vi "PH_SRDG645.evt Call Set Trigger.vi"(0 "i ref in":refnum<vi>, 2 "Generator Instance":string="N/A", 3 "Trigger Settings":T1={"Source"=0, "Rate [Hz]"=1000.0, "Level [V]"=1.0} {"Rate [Hz]" format="%#_9p"; "Source" items=["Internal", "External rising edge", "External falling edge", "Single shot external rising edges", "Single shot external falling edges", "Single shot", "Line"]}, 5 "error IO":errorcluster) -> (14 "i ref out":refnum<vi>, 19 "error out":errorcluster)   [LabVIEW 2014, in "PH_SRDG645.lvlib"]
doc: "This VI sends a simple event call."
uses:
  PH_SRDG645.lvlib
  PH_SRDG645.Trigger.ctl
  CS_Core/CSSystem/CoreLib/CoreLib.int 2 byte array.vi
  CS_Core/CSSystem/CoreLib/CoreLib.double 2 byte array.vi
  CS_Core/CSSystem/CoreLib/CoreLib.lvlib
  CS_Core/BaseProcess/BaseProcess.lvlib
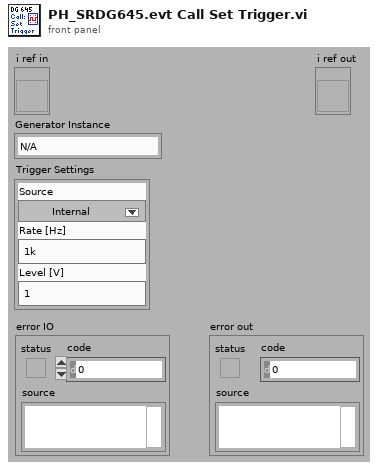
[diagram p1: front panel]
types:
  T1 = typedef "PH_SRDG645.lvlib/PH_SRDG645.Trigger.ctl" = cluster{"Source":i32, "Rate [Hz]":dbl, "Level [V]":dbl}
  T2 = typedef "CoreDefs.rawDataType.ctl" = i8[]
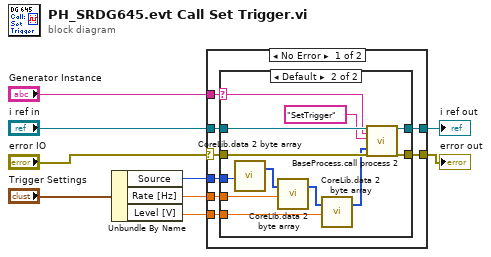
[diagram p0: block diagram]
diagram:
  n1 = Unbundle By Name("Trigger Settings") -> ("Source"=w3:i32, "Rate [Hz]"=w2:dbl, "Level [V]"=w1:dbl)
  n2 = case shown="No Error" "error IO" {
    selector: "error IO" -> [w17 w32]
    tunnel: "Generator Instance" -> [w10 _]
    tunnel: [w16 w32] -> w9
    tunnel: [w14 w33] -> w8
    tunnel: w1 -> [w11 _]
    tunnel: w2 -> [w12 _]
    tunnel: w3 -> [w13 _]
    tunnel: "i ref in" -> [w15 w33]
    frame No Error {
      n3 = case shown="Default" w10 {
        selector: w10 -> [_ w24]
        tunnel: w17 -> [w18 w31]
        tunnel: [w18 w30] -> w16
        tunnel: w15 -> [w19 w29]
        tunnel: [w19 w28] -> w14
        tunnel: w13 -> [_ w21]
        tunnel: w12 -> [_ w23]
        tunnel: w11 -> [_ w22]
        frame "", "N/A" {
        }
        frame Default {
          n4 = call-poly "CoreLib.data 2 byte array.vi"("i32"=w21) -> ("byteArray out"=w26:T2)  [unwired: 18 in]
          n5 = call-poly "CoreLib.data 2 byte array.vi"("byteArray"=w26, "f64"=w23) -> ("byteArray out"=w25:T2)  [unwired: 17 in]
          n6 = call-poly "CoreLib.data 2 byte array.vi"("byteArray"=w25, "f64"=w22) -> ("byteArray out"=w20:T2)  [unwired: 17 in]
          n7 = call "BaseProcess.call process 2.vi"("i ref in"=w29, "Object"=w24, "Selector"="SetTrigger", "Data"=w20, "error in (no error)"=w31) -> ("i ref out"=w28:refnum<vi>, "error out"=w30:errorcluster)  [unwired: 13 in]
        }
      }
    }
    frame Error {
    }
  }
  "error out" <- w9
  "i ref out" <- w8
